vi "PixyCam_SendWord.vi"(4 "error in":errorcluster, 6 "WriteWord":u16, 7 "PixyCamDevRef":T1) -> (0 "error out":errorcluster, 3 "PixyCamDevRef Out":T1)   [LabVIEW 2016, in "PixyCam_LabVIEW.lvlib"]
uses:
  PixyCam_LabVIEW.lvlib
  PixyCam_DevRef.ctl
  PixyCam_SPI_DevRef.ctl
  <vilib>/Rock Robotics/WPI/SPI/WPI_SPIDevRef.ctl
  <vilib>/Rock Robotics/SystemInterfaces/spilib/spi_bus.ctl
  PixyCam_CommMode.ctl
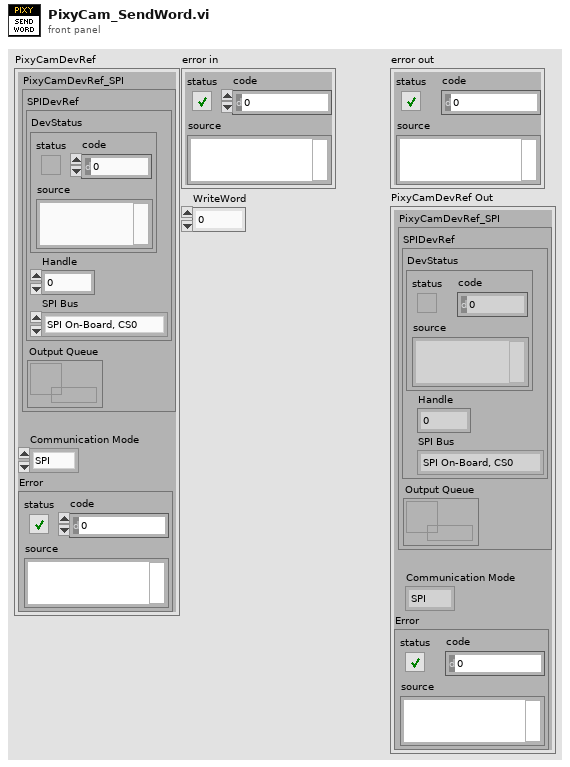
[diagram p1: front panel]
types:
  T1 = typedef "PixyCam_LabVIEW.lvlib/PixyCam_DevRef.ctl" = cluster{"PixyCamDevRef_SPI":T2, "Communication Mode":T5, "Error":errorcluster}
  T2 = typedef "PixyCam_LabVIEW.lvlib/PixyCam_SPI_DevRef.ctl" = cluster{"SPIDevRef":T3, "Output Queue":refnum<queue>}
  T3 = typedef "WPI_SPIDevRef.ctl" = cluster{"DevStatus":errorcluster, "Handle":i32, "SPI Bus":T4}
  T4 = typedef "spi_bus.ctl" = enum16{"SPI On-Board, CS0", "SPI On-Board, CS1", "SPI On-Board, CS2", "SPI On-Board, CS3", "SPI MXP", "Invalid"}
  T5 = typedef "PixyCam_LabVIEW.lvlib/PixyCam_CommMode.ctl" = enum16{"SPI", "I2C", "UART", "Analog", "Digital"}
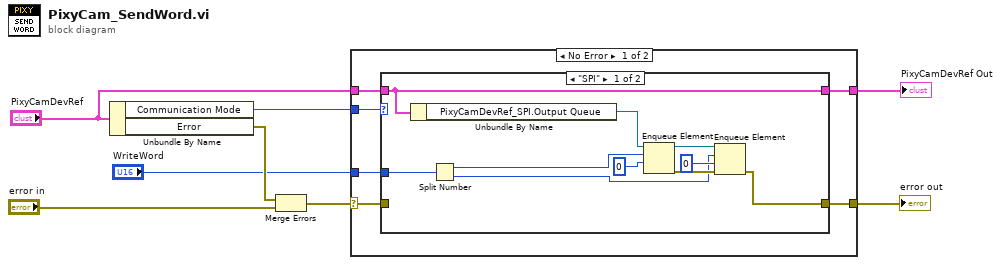
[diagram p0: block diagram]
diagram:
  n1 = Unbundle By Name("PixyCamDevRef") -> ("Communication Mode"=w4:T5, "Error"=w8:errorcluster)
  n2 = Merge Errors(w8, "error in") -> (w6:errorcluster)
  n3 = case shown="No Error" w6 {
    selector: w6 -> [w9 w28]
    tunnel: [w10 w28] -> w5
    tunnel: w4 -> [w14 _]
    tunnel: "PixyCamDevRef" -> [w13 w27]
    tunnel: [w12 w27] -> w2
    tunnel: "WriteWord" -> [w11 _]
    frame No Error {
      n4 = case shown="\"SPI\"" w14 {
        tunnel: w13 -> [w15 w26]
        tunnel: [w15 w26] -> w12
        tunnel: w11 -> [w19 _]
        tunnel: [w20 w25] -> w10
        tunnel: w9 -> [_ w25]
        frame "SPI" {
          n5 = Unbundle By Name(w15) -> ("PixyCamDevRef_SPI.Output Queue"=w24:refnum<queue>)
          n6 = Split Number(x=w19) -> (hi(x)=w18:u8, lo(x)=w16:u8)
          n7 = Enqueue Element(queue=w24, element=w18, timeout in ms (-1)=0) -> (queue out=w22:refnum<queue>, error out=w21:errorcluster)  [unwired: 1 in, 1 out]
          n8 = Enqueue Element(queue=w22, element=w16, timeout in ms (-1)=0, error in (no error)=w21) -> (error out=w20:errorcluster)  [unwired: 2 out]
        }
        frame Default {
        }
      }
    }
    frame Error {
    }
  }
  "error out" <- w5
  "PixyCamDevRef Out" <- w2
